vi "MakeSegmentUtility.vi"(0 "TreeNode DVR in":refnum<data-value>, 5 "DBL Array":sgl[](array[numeric]), 7 "Start time":sgl, 9 "dt":sgl, 11 "error in (no error)":errorcluster) -> (4 "TreeNode DVRout":refnum<data-value>, 15 "error out":errorcluster)   [LabVIEW 2012]
uses:
  <vilib>/MDSplus/Classes/Data_Class/TreeNode_Class/TreeNode.lvclass
  <vilib>/MDSplus/Library/MDSplus.lvlib
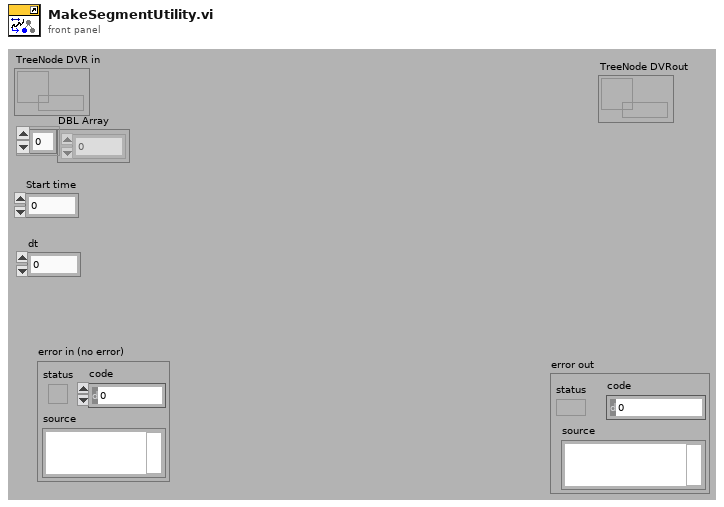
[diagram p1: front panel]
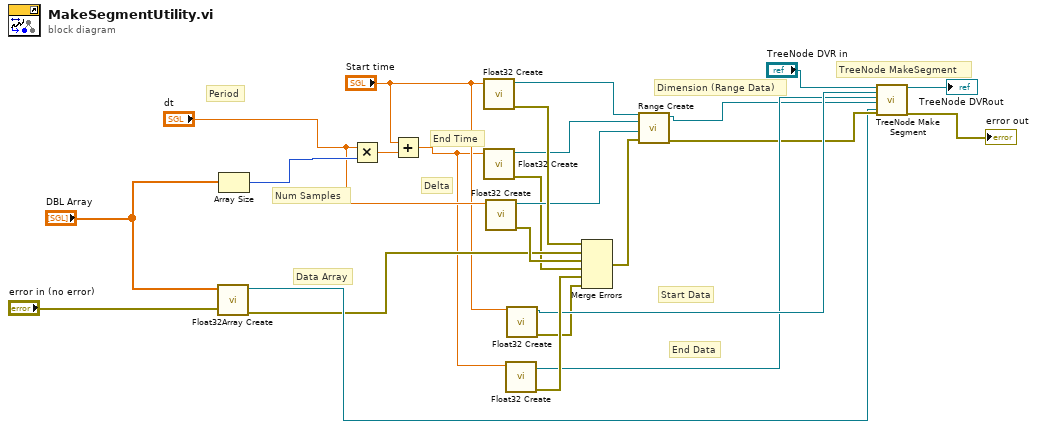
[diagram p0: block diagram]
diagram:
  # "TreeNode MakeSegment"
  # "Dimension (Range Data)"
  # "End Data"
  # "Start Data"
  # "Data Array"
  # "Delta"
  # "Num Samples"
  # "End Time"
  # "Period"
  n1 = call <vilib>:"Float32Array Create.vi"("error in (no error)"="error in (no error)", "SGL array in"="DBL Array") -> ("error out"=w9:errorcluster, "Float32Array DVR out"=w10:refnum<data-value>)  [unwired: 8 in]
  n2 = Array Size(array="DBL Array") -> (size(s)=w23:i32)
  n3 = Multiply(x="dt", y=w23) -> (x*y=w3:sgl)
  n4 = Add(x="Start time", y=w3) -> (x+y=w1:sgl)
  n5 = call <vilib>:"Float32 Create.vi"("SGL in"="Start time") -> ("error out"=w21:errorcluster, "Float32 DVR out"=w20:refnum<data-value>)  [unwired: 9 in]
  n6 = call <vilib>:"Float32 Create.vi"("SGL in"=w1) -> ("error out"=w6:errorcluster, "Float32 DVR out"=w19:refnum<data-value>)  [unwired: 9 in]
  n7 = call <vilib>:"Float32 Create.vi"("SGL in"="dt") -> ("error out"=w22:errorcluster, "Float32 DVR out"=w18:refnum<data-value>)  [unwired: 9 in]
  n8 = call <vilib>:"Float32 Create.vi"("SGL in"=w1) -> ("error out"=w16:errorcluster, "Float32 DVR out"=w13:refnum<data-value>)  [unwired: 9 in]
  n9 = call <vilib>:"Float32 Create.vi"("SGL in"="Start time") -> ("error out"=w5:errorcluster, "Float32 DVR out"=w14:refnum<data-value>)  [unwired: 9 in]
  n10 = Merge Errors(w21, w9, w22, w6, w16, w5) -> (w17:errorcluster)
  n11 = call <vilib>:"Range Create.vi"("error in (no error)"=w17, "Delta value"=w18, "Ending"=w19, "Begin"=w20) -> ("error out"=w11:errorcluster, "Range DVR out"=w12:refnum<data-value>)  [unwired: 6 in]
  n12 = call <vilib>:"TreeNode Make Segment.vi"("TreeNode DVR in"="TreeNode DVR in", "Start"=w14, "End"=w13, "Dimension"=w12, "Data"=w10, "error in (no error)"=w11) -> ("TreeNode DVR out"=→"TreeNode DVRout":refnum<data-value>, "error out"=→"error out":errorcluster)  [unwired: 12 in]
